vi "Do.vi"(8 "error in (no error)":errorcluster, 10 "Actor in":refnum<class "Actor.lvclass">, 11 "Move Msg":refnum<class "Move Msg.lvclass">) -> (0 "error out":errorcluster, 2 "Actor out":refnum<class "Actor.lvclass">)   [LabVIEW 2016, in "CS++Motor.lvlib" / "Move Msg.lvclass"]
doc: "This VI delivers the message to the actor by calling the appropriate method(s) on the actor."
uses:
  Move Msg.lvclass
  <vilib>/ActorFramework/Actor/Actor.lvclass
  C:/User/Brand/LVP/CSPP-Dev/Packages/CSPP_Core/Actors/CS++PVMonitor Messages/CS++PVUpdate Msg/CS++PVUpdate Msg.lvclass
  CS++Motor/CS++Motor.lvclass
  C:/Program Files (x86)/National Instruments/LabVIEW 2016/vi.lib/ActorFramework/Actor/Actor.lvclass
  CSPP_Core/Actors/CS++PVMonitor Messages/CS++PVUpdate Msg/CS++PVUpdate Msg.lvclass/CS++PVUpdate Msg.ctl
  CSPP_Core/Classes/CS++ProcessVariables/ProcessVariable/PV.lvclass/PV.ctl
  Move Msg.lvclass/Move Msg.ctl
  CSPP_Core/Classes/CS++ProcessVariables/ProcessVariable/PV.lvclass
  CSPP_Core/Actors/CS++PVMonitor Messages/CS++PVUpdate Msg/CS++PVUpdate Msg.lvclass
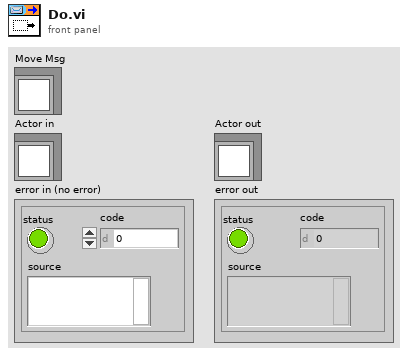
[diagram p1: front panel]
types:
  T1 = cluster{"AxisNumber":u8, "Position":dbl, "Relative?":bool}
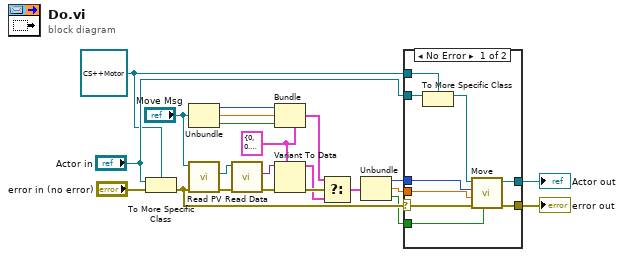
[diagram p0: block diagram]
diagram:
  w14 = T1 {"AxisNumber"=0, "Position"=0.0, "Relative?"=FALSE} ("Type")
  w18 = refnum<class "CS++Motor.lvclass"> refnum ("Actor in")
  n1 = To More Specific Class(target class=w18, reference="Actor in", error in="error in (no error)") -> (error out=w7:errorcluster)  [unwired: 1 out]
  n2 = Unbundle ("Pre-Unbundler")("Move Msg") -> (w3:u8, w2:dbl, w1:bool)
  n3 = call "Read PV.vi"("error in (no error)"=w7, "CS++PVUpdate Msg in"="Move Msg") -> ("error out"=w17:errorcluster, "PV"=w13:refnum<class "PV.lvclass">)  [unwired: 7 in, 1 out]
  n4 = call "Read Data.vi"("error in (no error)"=w17, "PV in"=w13) -> ("error out"=w11:errorcluster, "Data"=w12:variant)  [unwired: 7 in, 1 out]
  n5 = Bundle ("Pre-Bundler")(cluster=w14, "AxisNumber"=w3, "Position"=w2, "Relative?"=w1) -> (w15:T1)
  n6 = Variant To Data(error in=w11, type=w14, Variant=w12) -> (data=w9:T1, error out=w16:errorcluster)
  n7 = Select ("MainSelect")(t=w15, s=w16, f=w9) -> (s? t:f=w10:T1)
  n8 = Unbundle ("Main-Unbundler")(w10) -> ("AxisNumber"=w6:u8, "Position"=w5:dbl, "Relative?"=w4:bool)
  n9 = case shown="No Error" w7 {
    selector: w7 -> [w29 w33]
    tunnel: [w31 w33] -> w21
    tunnel: [w30 w32] -> w20
    tunnel: "Actor in" -> [w28 w32]
    tunnel: w18 -> [w27 _]
    tunnel: w6 -> [w25 _]
    tunnel: w5 -> [w24 _]
    tunnel: w4 -> [w23 _]
    frame No Error {
      n10 = To More Specific Class(target class=w27, reference=w28) -> (specific class reference=w26:refnum<class "CS++Motor.lvclass">)  [unwired: 1 in, 1 out]
      n11 = call "Move.vi"("Relative?"=w23, "error in (no error)"=w29, "SetPosition"=w24, "AxisNumber"=w25, "CS++Motor in"=w26) -> ("error out"=w31:errorcluster, "CS++Motor out"=w30:refnum<class "CS++Motor.lvclass">)  [unwired: 5 in]
    }
    frame Error {
    }
  }
  "error out" <- w21
  "Actor out" <- w20
